vi "Cannon Arming.vi"(1 "Cannon Info In":T2) -> (0 "Cannon Info Out":T2)   [LabVIEW 2013]
uses:
  <vilib>/Rock Robotics/WPI/Relay/WPI_RelayValue.ctl
  Cannon Global.vi
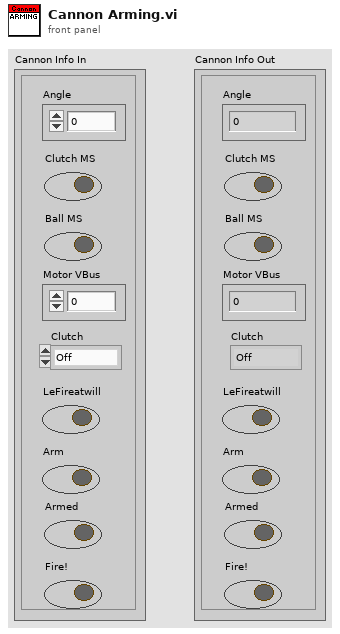
[diagram p1: front panel]
types:
  T1 = typedef "WPI_RelayValue.ctl" = enum16{"Off", "On", "Forward", "Reverse"}
  T2 = cluster{"Angle":dbl, "Clutch MS":bool, "Ball MS":bool, "Motor VBus":dbl, "Clutch ":T1, "LeFireatwill":bool, "Arm":bool, "Armed":bool, "Fire!":bool}
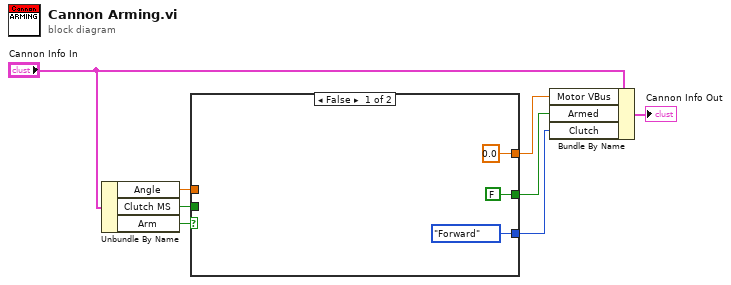
[diagram p0: block diagram]
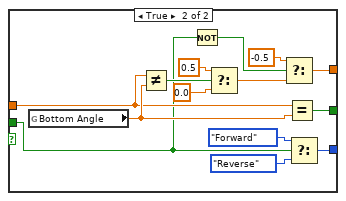
[diagram p2: hidden frame]
diagram:
  n1 = Unbundle By Name("Cannon Info In") -> ("Angle"=w5:dbl, "Clutch MS"=w4:bool, "Arm"=w3:bool)
  n2 = case shown="False" w3 {
    tunnel: [0.0 w22] -> w6
    tunnel: w5 -> [_ w18]
    tunnel: w4 -> [_ w14]
    tunnel: [FALSE w17] -> w2
    tunnel: [WPI_RelayValue."Forward" ("Clutch") w15] -> w1
    frame False {
    }
    frame True {
      n3 = global read "Cannon Global.vi" "Bottom Angle"() -> (w19:dbl)
      n4 = Not Equal?(x=w18, y=w19) -> (x != y?=w16:bool)
      n5 = Not(x=w14) -> (.not. x?=w25:bool)
      n6 = Select(t=0.5, s=w16, f=0.0) -> (s? t:f=w23:dbl)
      n7 = Select(t=-0.5, s=w25, f=w23) -> (s? t:f=w22:dbl)
      n8 = Equal?(x=w18, y=w19) -> (x = y?=w17:bool)
      n9 = Select(t=WPI_RelayValue."Forward" ("Clutch"), s=w14, f=WPI_RelayValue."Reverse" ("Clutch")) -> (s? t:f=w15:T1)
    }
  }
  n10 = Bundle By Name(cluster="Cannon Info In", "Motor VBus"=w6, "Armed"=w2, "Clutch"=w1) -> (→"Cannon Info Out":T2)
